vi "Panel.vi"(11 "Dashboard Panel in":refnum<class "Dashboard Panel.lvclass">) -> ()   [LabVIEW 2020, in "SB App.lvlib" / "Dashboard Panel.lvclass"]
uses:
  Dashboard Panel.lvclass
  C:/Program Files (x86)/National Instruments/LabVIEW 2020/vi.lib/IlluminatedG/IG OOPanel/OOPanel/Panel/Panel.lvclass
  <vilib>/IlluminatedG/IG OOPanel/OOPanel/Panel/Basic UI State.ctl
  Dashboard Panel.lvclass/Dashboard Panel.ctl
  <vilib>/IlluminatedG/IG OOPanel/OOPanel/Panel/Panel.lvclass
  <vilib>/IlluminatedG/IG OOPanel/OOPanel/OOPanel.lvlib
panel:
  out "Round":u32
  in  "Stop":bool
  in  "Step":bool
  in  "Start":bool
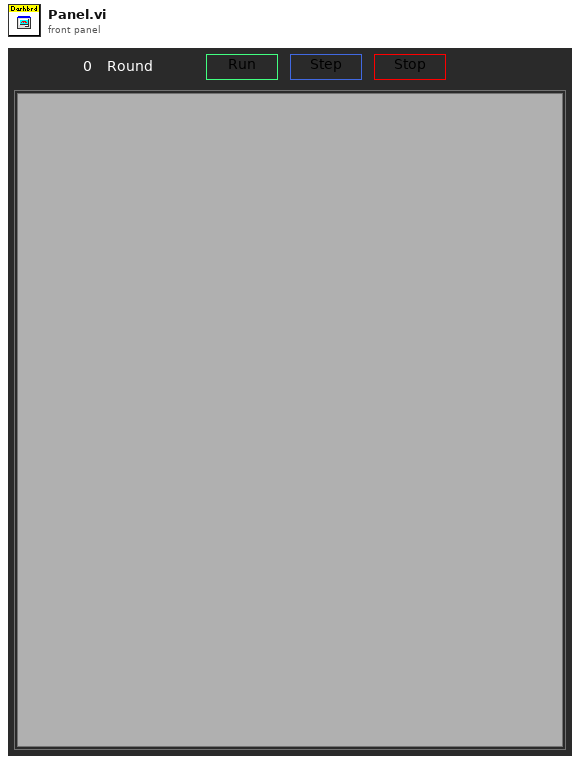
[diagram p1: front panel]
types:
  T1 = typedef "OOPanel.lvlib/Panel.lvclass/Basic UI State.ctl" = enum16{"Init", "Run", "Close"}
  T2 = enum8{"Enabled", "Disabled", "Disabled and Grayed Out"}
  T3 = typedef "SB App.lvlib/Dashboard Panel.lvclass/Incoming Events.ctl" = cluster{"Round":refnum<user-event>}
  T4 = typedef "OOPanel.lvlib/Panel.lvclass/Panel Events.ctl" = cluster{"Visbility":refnum<user-event>, "Close":refnum<user-event>}
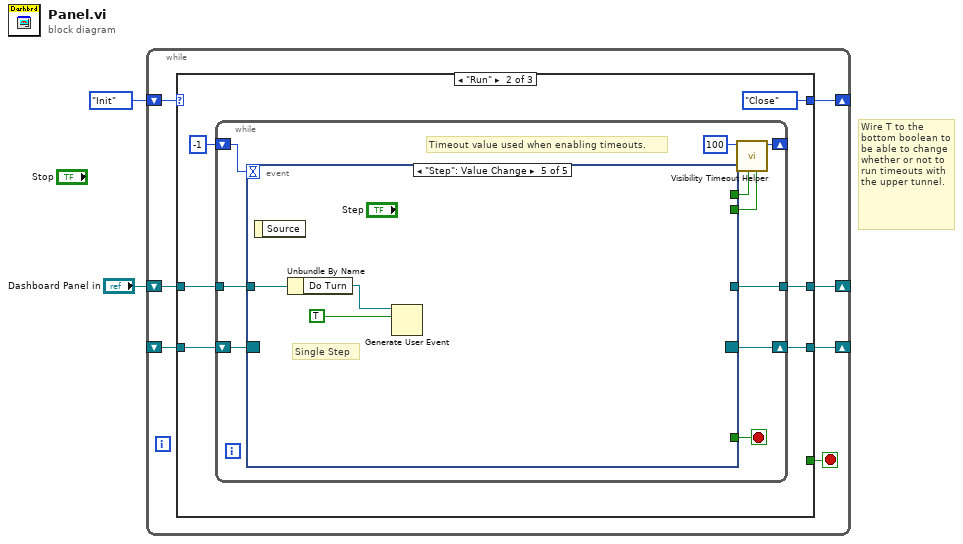
[diagram p0: block diagram]
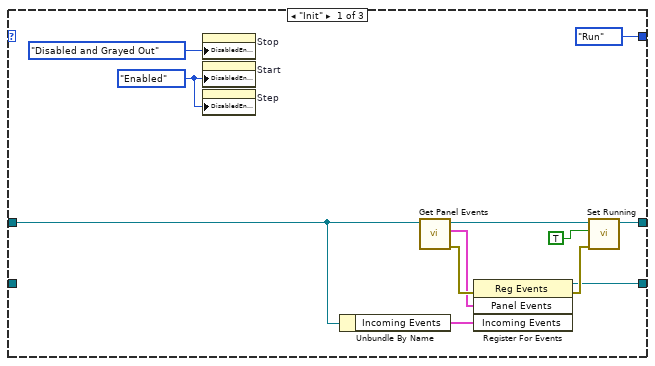
[diagram p2: hidden frame]
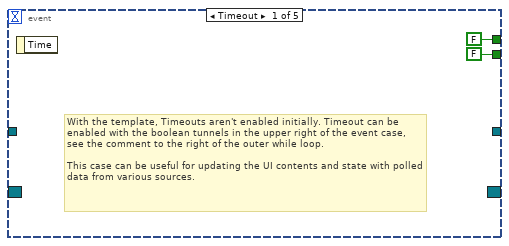
[diagram p3: hidden frame]
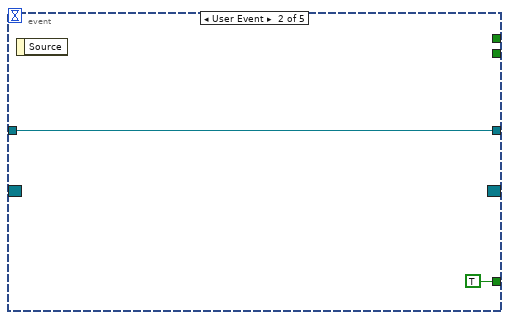
[diagram p4: hidden frame]
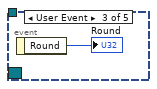
[diagram p5: hidden frame]
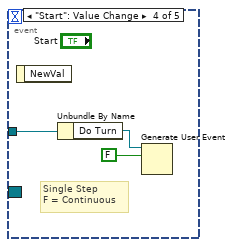
[diagram p6: hidden frame]
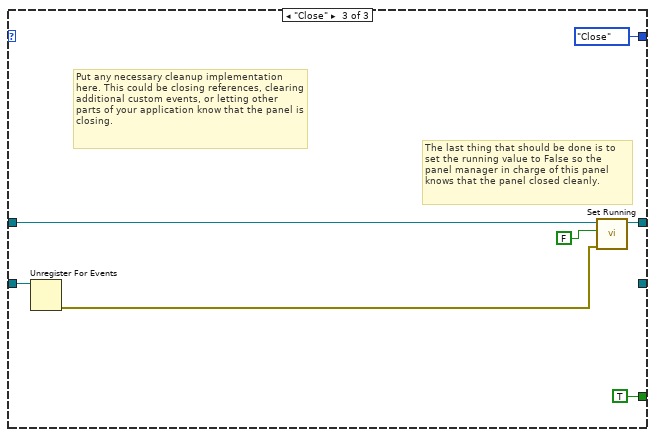
[diagram p7: hidden frame]
diagram:
  # "Wire T to the bottom boolean to be able to change whether or not to run timeouts with the upper tunnel."
  n1 = while {
    shift-right: [w8] -> _
    shift-left: _ -> [w9]
    shift-right: [w6] -> _
    shift-left: Basic_UI_State."Init" ("Basic UI State") -> [w7]
    shift-right: [w4] -> _
    shift-left: "Dashboard Panel in" -> [w3]
    stop <- w5 stop-if-true
    n2 = case shown="\"Run\"" w7 {
      tunnel: w9 -> [_ w27 w51]
      tunnel: [w15 w25 _] -> w8
      tunnel: [Basic_UI_State."Run" ("Basic UI State") Basic_UI_State."Close" ("Basic UI State") Basic_UI_State."Close" ("Basic UI State")] -> w6
      tunnel: [_ _ TRUE] -> w5
      tunnel: [w14 w22 w49] -> w4
      tunnel: w3 -> [w11 w23 w50]
      frame "Init" {
        w12 = T2."Enabled" ("Disabled")
        n3 = property on="Stop" class="Bool"("DisabledEnum"=T2."Disabled and Grayed Out" ("Disabled")) -> ()  [unwired: 2 in, 2 out]
        n4 = property on="Start" class="Bool"("DisabledEnum"=w12) -> ()  [unwired: 2 in, 2 out]
        n5 = property on="Step" class="Bool"("DisabledEnum"=w12) -> ()  [unwired: 2 in, 2 out]
        n6 = Unbundle By Name(w11) -> ("Incoming Events"=w10:T3)
        n7 = call <vilib>:"Get Panel Events.vi"("Panel in"=w11) -> ("error out"=w21:errorcluster, "Panel Events"=w17:T4, "Panel out"=w18:refnum<class "Dashboard Panel.lvclass">)  [unwired: 8 in]
        n8 = register-events(error in=w21, w17, w10) -> (reference out=w15:refnum<event-registration>, error out=w19:errorcluster)  [unwired: 1 in]
        n9 = call <vilib>:"Set Running.vi"("error in (no error)"=w19, "Running"=TRUE, "Panel in"=w18) -> ("Panel out"=w14:refnum<class "Dashboard Panel.lvclass">)  [unwired: 7 in, 1 out]
      }
      frame "Run" {
        n10 = while {
          shift-right: [w33] -> w25
          shift-left: w27 -> [w34]
          shift-right: [w36] -> _
          shift-left: -1 ("Timeout") -> [w35]
          tunnel: w23 -> [w29]
          tunnel: [w28] -> w22
          stop <- w30 stop-if-true
          # "Timeout value used when enabling timeouts."
          n11 = event shown="[4] \"Step\": Value Change" {
            selector: w34 -> [_ _ _ _ _]
            dyn-events: [_ _ _ _ _] -> w33
            timeout: w35 -> [_ _ _ _ _]
            tunnel: [FALSE _ _ _ _] -> w32
            tunnel: [FALSE _ _ _ _] -> w31
            tunnel: [_ TRUE _ _ _] -> w30
            tunnel: w29 -> [_ w40 _ w45 w48]
            tunnel: [_ w40 _ _ _] -> w28
            event Timeout {
              # "With the template, Timeouts aren't enabled initially. Timeout can be enabled with the boolean tunnels in the upper right of the event case, see the comment to the right of the outer while loop.\n\nThis case can be useful for updating the UI contents and state with polled data from various sources."
              n12 = event-data() -> ()  [unwired: 1 in, 1 out]
            }
            event User Event {
              n13 = event-data() -> ()  [unwired: 1 in, 1 out]
            }
            event User Event {
              n14 = event-data() -> ("Round"=→"Round":u32)  [unwired: 1 in]
            }
            event "Start": Value Change {
              # "Single Step\nF = Continuous"
              n15 = event-data() -> ()  [unwired: 1 in, 1 out]
              n16 = Unbundle By Name(w45) -> ("Do Turn"=w44:refnum<user-event>)
              n17 = Generate User Event(user event=w44, event data cluster=FALSE ("event data")) -> ()  [unwired: 2 in, 2 out]
            }
            event "Step": Value Change {
              # "Single Step"
              n18 = event-data() -> ()  [unwired: 1 in, 1 out]
              n19 = Unbundle By Name(w48) -> ("Do Turn"=w47:refnum<user-event>)
              n20 = Generate User Event(user event=w47, event data cluster=TRUE ("event data")) -> ()  [unwired: 2 in, 2 out]
            }
          }
          n21 = call <vilib>:"Visibility Timeout Helper.vi"("Update?"=w31, "Use Timeout?"=w32, "Visible Timeout mS"=100) -> ("Timeout"=w36:i32)  [unwired: 8 in]
        }
      }
      frame "Close" {
        # "Put any necessary cleanup implementation here. This could be closing references, clearing additional custom events, or letting other parts of your application know that the panel is closing."
        # "The last thing that should be done is to set the running value to False so the panel manager in charge of this panel knows that the panel closed cleanly."
        n22 = Unregister For Events(event registration refnum=w51) -> (error out=w53:errorcluster)  [unwired: 1 in]
        n23 = call <vilib>:"Set Running.vi"("error in (no error)"=w53, "Running"=FALSE, "Panel in"=w50) -> ("Panel out"=w49:refnum<class "Dashboard Panel.lvclass">)  [unwired: 7 in, 1 out]
      }
    }
  }
